vi "SetPersistentConfiguration.vi"(8 "ErrorIn":errorcluster, 9 "DataIn":variant, 11 "ObjectIn":refnum<class "YAFTAF.lvclass">) -> (0 "ErrorOut":errorcluster, 1 "DataOut":variant, 3 "ObjectOut":refnum<class "YAFTAF.lvclass">)   [LabVIEW 2021, in "YAFTAF.lvclass"]
uses:
  YAFTAF.lvclass
  C:/Localdata/Projects/TriekselSoft/TriekselsoftApplicationFramework/Source/.Externals/Library_YAF/YActor/YActor.lvclass
  YActor/YActor.lvclass/YActor.ctl
  YActor/ExeCmd_sync.vi
  YActor/private/SendCommand.vi
  YActor/private/WaitForReply.vi
  YActor/private/CreateLocalVI.vi
  YActor/private/ExeuteInlineVI.vi
  YActor/private/GetRemoteVIRef.vi
  YActor/private/GetNameOfVI.vi
  YActor/QuickCast.vi
  YActor/private/VINameProperty.vi
  YActor/private/MessageCounter.vi
  YActor/InlineReferencePool.vi
  YActor/private/ExecuteVI.vi
  YActor/YActor.lvclass
  YAFTAF.lvclass/YAFTAF.ctl
  C:/Localdata/Projects/TriekselSoft/TriekselsoftApplicationFramework/Source/.Externals/Interface_UserInterface_IFrontPanel/IFrontPanel/IFrontPanel.lvclass
  C:/Localdata/Projects/TriekselSoft/TriekselsoftApplicationFramework/Source/IInterface/IInterface.lvclass
  C:/Localdata/Projects/TriekselSoft/TriekselsoftApplicationFramework/Source/.Externals/Interface_Object_ICreateDestroy/ICreateDestroy/ICreateDestroy.lvclass
  C:/Localdata/Projects/TriekselSoft/TriekselsoftApplicationFramework/Source/.Externals/Interface_Object_IPersistentData/IPersistentData/IPersistentData.lvclass
  C:/Localdata/Projects/TriekselSoft/TriekselsoftApplicationFramework/Source/.Externals/Interface_TAF_ITAFObject/ITAFObject/ITAFObject.lvclass
  C:/Localdata/Projects/TriekselSoft/TriekselsoftApplicationFramework/Source/.Externals/Library_YAF/YAFTAF/YAFTAF.lvclass
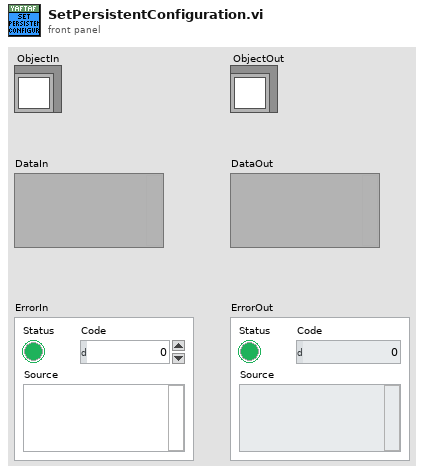
[diagram p1: front panel]
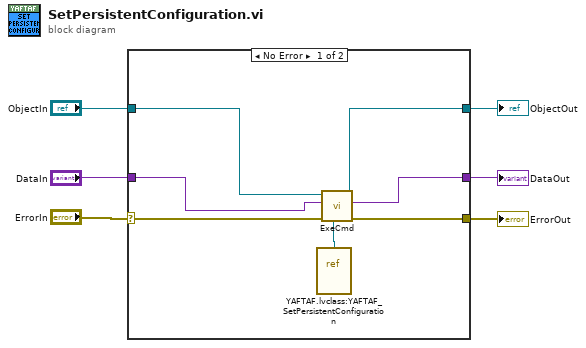
[diagram p0: block diagram]
diagram:
  n1 = case shown="No Error" "ErrorIn" {
    selector: "ErrorIn" -> [w12 w16]
    tunnel: [w13 w16] -> w6
    tunnel: [w10 w15] -> w3
    tunnel: "ObjectIn" -> [w8 w15]
    tunnel: "DataIn" -> [w7 w14]
    tunnel: [w9 w14] -> w2
    frame No Error {
      n2 = vi-ref "YAFTAF.lvclass:YAFTAF_SetPersistentConfiguration.vi"() -> (w11:refnum<vi>)
      n3 = call-poly "ExeCmd.vi"("CmdVIRef"=w11, "ErrorIn"=w12, "CmdData"=w7, "YActorIn"=w8) -> ("ErrorOut"=w13:errorcluster, "ReplyData"=w9:variant, "YActorOut"=w10:refnum<class "YAFTAF.lvclass">)  [unwired: 5 in]
    }
    frame Error {
    }
  }
  "ErrorOut" <- w6
  "ObjectOut" <- w3
  "DataOut" <- w2
